vi "Read Context I32 1.vi"(8 "error in (no error)":errorcluster, 11 "Context in":refnum<class "Context.lvclass">) -> (0 "error out":errorcluster, 2 "Context I32":i32, 3 "Context out":refnum<class "Context.lvclass">)   [LabVIEW 2021, in "Context.lvclass"]
uses:
  Context.lvclass
  Context.lvclass/Context.ctl
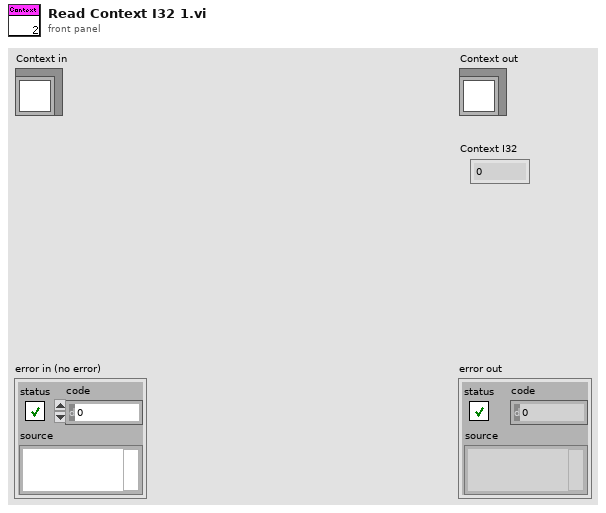
[diagram p1: front panel]
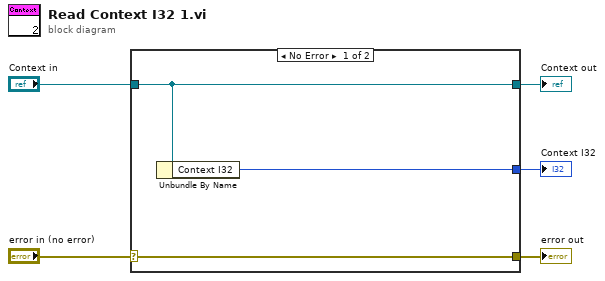
[diagram p0: block diagram]
diagram:
  n1 = case shown="No Error" "error in (no error)" {
    selector: "error in (no error)" -> [w8 w9]
    tunnel: [w8 w9] -> w4
    tunnel: [w7 w10] -> w2
    tunnel: "Context in" -> [w7 w10]
    tunnel: [w6 _] -> w1
    frame No Error {
      n2 = Unbundle By Name(w7) -> ("Context I32"=w6:i32)
    }
    frame Error {
    }
  }
  "error out" <- w4
  "Context out" <- w2
  "Context I32" <- w1
